vi "LWXPS_PositionerCompensationSpatialPeriodicNotchsGet.vi"(0 "XPS Reference IN":refnum<k24>, 2 "Positioner Name":string, 5 "LabVIEW error IN":errorcluster) -> (7 "LabVIEW error OUT":errorcluster, 8 "XPS Reference OUT":refnum<k24>, 9 "XPS Error String":string, 10 "Returned error code":i32, 11 "Spatial Notch Gain 3":dbl, 12 "Spatial Notch Step 1":dbl, 13 "Spatial Notch Bandwidth 3":dbl, 14 "Spatial Notch Bandwidth 1":dbl, 15 "Spatial Notch Gain 1":dbl, 16 "Spatial Notch Step 2":dbl, 17 "Spatial Notch Bandwidth 2":dbl, 18 "Spatial Notch Gain 2":dbl, 19 "Spatial Notch Step 3":dbl)   [LabVIEW 2014]
uses:
  D:/XPSQ8_LabView_Library/Development/Source/Dll/Newport.XPS.CommandInterface.dll
  Dll/Newport.XPS.CommandInterface.dll
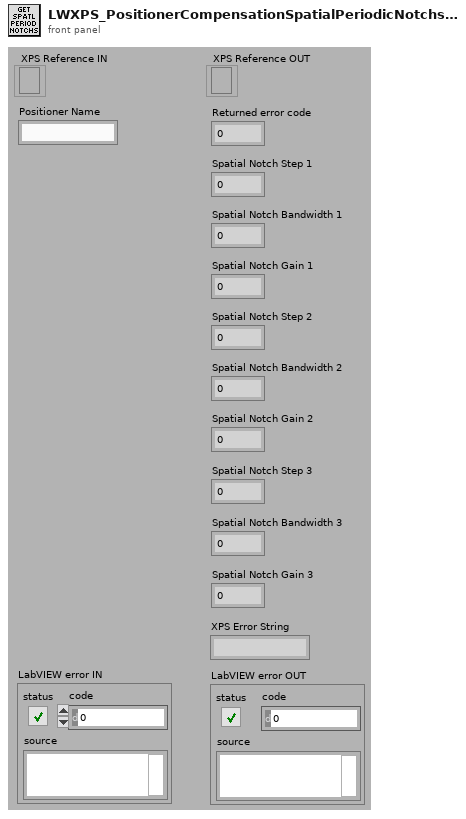
[diagram p1: front panel]
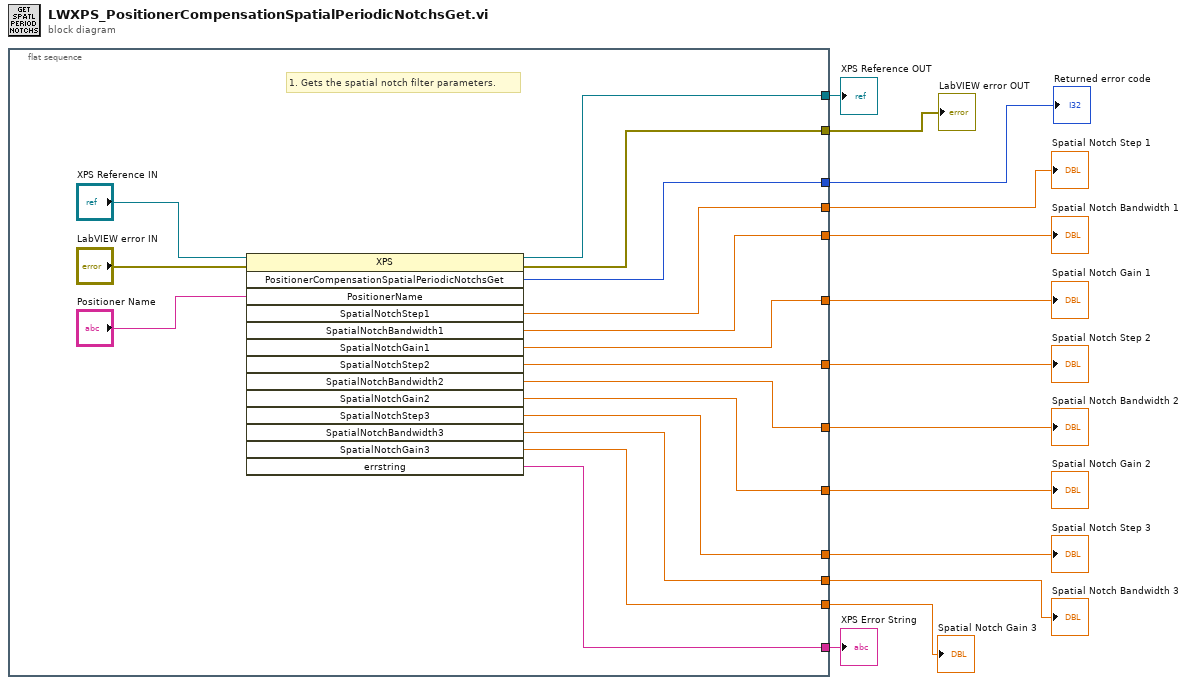
[diagram p0: block diagram]
diagram:
  n1 = flat-sequence {
    tunnel: [w27] -> w13
    tunnel: [w24] -> w12
    tunnel: [w28] -> w11
    tunnel: [w19] -> w10
    tunnel: [w22] -> w9
    tunnel: [w23] -> w6
    tunnel: [w21] -> w8
    tunnel: [w20] -> w7
    tunnel: [w18] -> w5
    tunnel: [w17] -> w4
    tunnel: [w16] -> w3
    tunnel: [w15] -> w2
    tunnel: [w14] -> w1
    frame #0 {
      # "1. Gets the spatial notch filter parameters."
      n2 = invoke class="XPS" method="PositionerCompensationSpatialPeriodicNotchsGet"(reference="XPS Reference IN", error in="LabVIEW error IN", "PositionerName"="Positioner Name") -> (reference out=w27:refnum<k24>, error out=w24:errorcluster, "PositionerCompensationSpatialPeriodicNotchsGet"=w28:i32, "SpatialNotchStep1"=w19:dbl, "SpatialNotchBandwidth1"=w22:dbl, "SpatialNotchGain1"=w21:dbl, "SpatialNotchStep2"=w20:dbl, "SpatialNotchBandwidth2"=w23:dbl, "SpatialNotchGain2"=w18:dbl, "SpatialNotchStep3"=w17:dbl, "SpatialNotchBandwidth3"=w16:dbl, "SpatialNotchGain3"=w15:dbl, "errstring"=w14:string)  [unwired: 11 in, 1 out]
    }
  }
  "XPS Error String" <- w1
  "XPS Reference OUT" <- w13
  "LabVIEW error OUT" <- w12
  "Returned error code" <- w11
  "Spatial Notch Step 1" <- w10
  "Spatial Notch Bandwidth 1" <- w9
  "Spatial Notch Gain 1" <- w8
  "Spatial Notch Step 2" <- w7
  "Spatial Notch Bandwidth 2" <- w6
  "Spatial Notch Gain 2" <- w5
  "Spatial Notch Step 3" <- w4
  "Spatial Notch Bandwidth 3" <- w3
  "Spatial Notch Gain 3" <- w2
